vi "test.OutputBufferr.vi"() -> ()   [LabVIEW 2014]
uses:
  Private/Class/meth.Constructor.vi
  Private/Class/meth.SetStreamReader.vi
  Private/Class/meth.Destructor.vi
  GLue.lvlib
panel:
  out "Numeric":i32
  in  "Boolean":bool
  out "error out":errorcluster
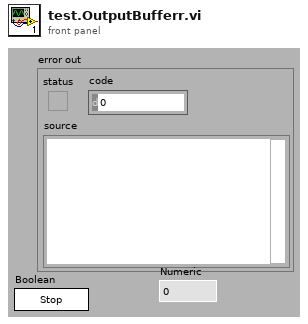
[diagram p1: front panel]
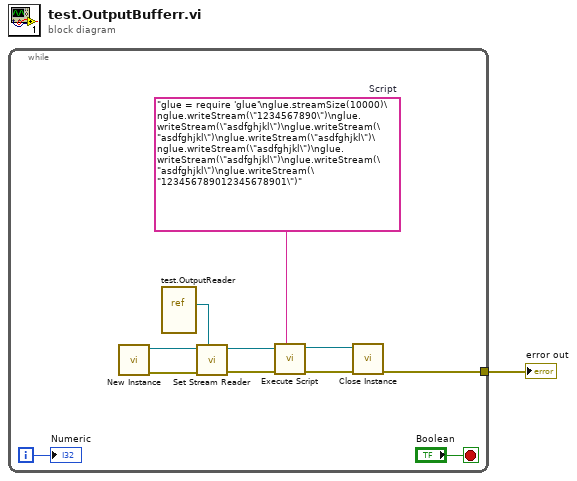
[diagram p0: block diagram]
diagram:
  n1 = while {
    tunnel: [w9] -> w1
    i -> [w2]
    stop <- "Boolean" stop-if-true
    w10 = "glue = require 'glue'\nglue.streamSize(10000)\nglue.writeStream(\"1234567890\")\nglue.writeStream(\"asdfghjkl\")\nglue.writeStream(\"asdfghjkl\")\nglue.writeStream(\"asdfghjkl\")\nglue.writeStream(\"asdfghjkl\")\nglue.writeStream(\"asdfghjkl\")\nglue.writeStream(\"asdfghjkl\")\nglue.writeStream(\"123456789012345678901\")"  # Script
    n2 = call "New Instance.vi"() -> ("error out"=w8:errorcluster, "GLue out"=w7:refnum<class "class.GLue.lvclass">)  [unwired: 10 in]
    n3 = vi-ref "test.OutputReader.vi"() -> (w4:refnum<vi>)
    n4 = call "Set Stream Reader.vi"("StreamReader"=w4, "error in"=w8, "GLue in"=w7) -> ("error out"=w5:errorcluster, "GLue out"=w6:refnum<class "class.GLue.lvclass">)  [unwired: 7 in]
    n5 = call "Execute Script.vi"("Script"=w10, "error in"=w5, "GLue in"=w6) -> ("error out"=w12:errorcluster, "GLue out"=w11:refnum<class "class.GLue.lvclass">)  [unwired: 6 in, 1 out]
    n6 = call "Close Instance.vi"("error in"=w12, "GLue in"=w11) -> ("error out"=w9:errorcluster)  [unwired: 9 in]
    "Numeric" <- w2
  }
  "error out" <- w1
